vi "DAQ_daqmxorg.vi"() -> ()   [LabVIEW 2020]
uses:
  <vilib>/Utility/error.llb/DialogType.ctl
  <vilib>/DAQmx/read.llb/DAQmx Read (Analog 2D DBL NChan NSamp).vi
  <vilib>/DAQmx/create/channels.llb/DAQmx Create Channel (AI-Voltage-Basic).vi
  <vilib>/DAQmx/configure/timing.llb/DAQmx Timing (Sample Clock).vi
  <vilib>/DAQmx/configure/trigger.llb/DAQmx Start Trigger (None).vi
  <vilib>/DAQmx/miscellaneous.llb/DAQmx Fill In Error Info.vi
panel:
  out "Waveform Chart 2":dbl[][](graph)
  out "data":dbl[][](array[numeric]) format="%0.2f"
  out "Boolean":bool
  in  "stop":bool
  out "Waveform Chart":dbl[][](graph)
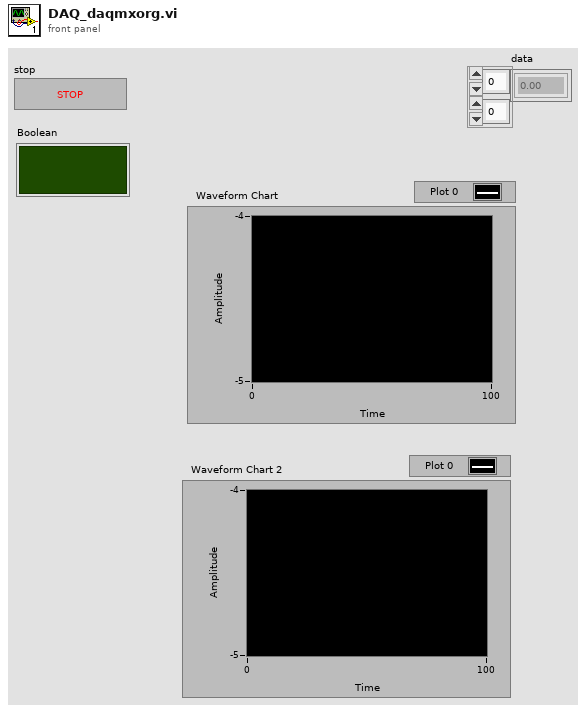
[diagram p1: front panel]
types:
  T1 = typedef "DialogType.ctl" = u16
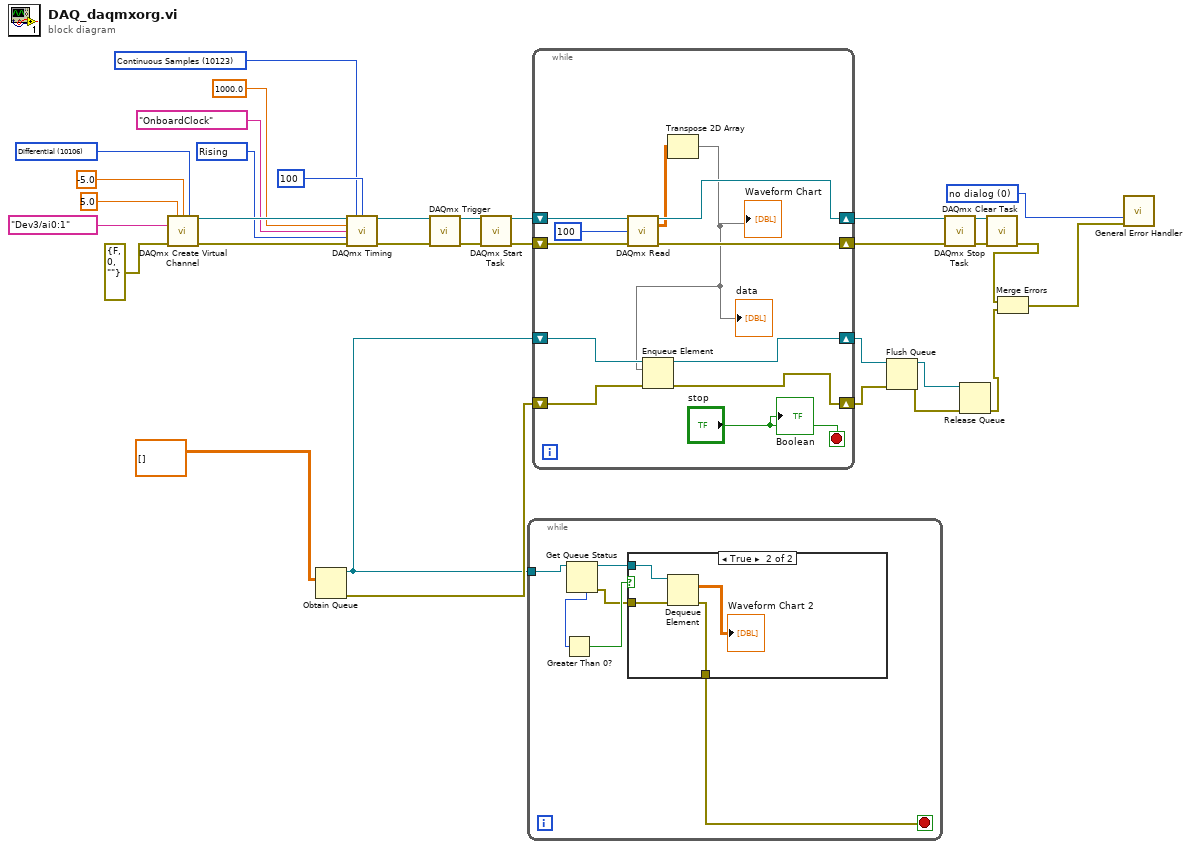
[diagram p0: block diagram]
diagram:
  w11 = T1 0 items=["no dialog", "OK message", "continue or stop message", "OK message + warnings", "continue/stop + warnings"] ("type of dialog (OK msg:1)")
  w22 = 10280 items=["Rising"=10280, "Falling"=10171] ("active edge")
  w25 = 10123 items=["Finite Samples"=10178, "Continuous Samples"=10123, "Hardware Timed Single Point"=12522] ("sample mode")
  w33 = 10106 items=["Default"=-1, "RSE"=10083, "NRSE"=10078, "Differential"=10106, "Pseudodifferential"=12529] ("input terminal configuration")
  n1 = call-poly <vilib>:"DAQmx Create Virtual Channel.vi"("maximum value"=5.0, "minimum value"=-5.0, "input terminal configuration"=w33, "physical channels"=tag "Dev3/ai0:1", "error in"=errorcluster {"status"=FALSE, "code"=0, "source"=""}) -> ("task out"=w27:refnum<k21>, "error out"=w28:errorcluster)  [unwired: 9 in]
  n2 = Obtain Queue(element data type=dbl[][] []) -> (queue out=w6:refnum<queue>, error out=w9:errorcluster)  [unwired: 4 in, 1 out]
  n3 = call-poly <vilib>:"DAQmx Timing.vi"("task/channels in"=w27, "sample mode"=w25, "samples per channel"=100, "rate"=1000.0, "source"=tag "OnboardClock", "active edge"=w22, "error in"=w28) -> ("task out"=w20:refnum<k21>, "error out"=w21:errorcluster)  [unwired: 7 in]
  n4 = call-poly <vilib>:"DAQmx Trigger.vi"("task/channels in"=w20, "error in"=w21) -> ("task out"=w19:refnum<k21>, "error out"=w18:errorcluster)  [unwired: 12 in]
  n5 = call <vilib>:"DAQmx Start Task.vi"("task/channels in"=w19, "error in"=w18) -> ("task out"=w17:refnum<k21>, "error out"=w16:errorcluster)  [unwired: 12 in]
  n6 = while {
    tunnel: w6 -> [w37]
    stop <- w35 stop-if-true
    n7 = Get Queue Status(queue=w37) -> (queue out=w36:refnum<queue>, error out=w34:errorcluster, # elements in queue=w39:i32)  [unwired: 2 in, 5 out]
    n8 = Greater Than 0?(x=w39) -> (x > 0?=w38:bool)
    n9 = case shown="True" w38 {
      tunnel: w36 -> [_ w44]
      tunnel: [w40 w43] -> w35
      tunnel: w34 -> [w40 w42]
      frame False {
      }
      frame True {
        n10 = Dequeue Element(queue=w44, error in (no error)=w42) -> (element=→"Waveform Chart 2":dbl[][], error out=w43:errorcluster)  [unwired: 1 in, 2 out]
      }
    }
  }
  n11 = while {
    shift-right: [w54] -> w15
    shift-left: w17 -> [w56]
    shift-right: [w53] -> w14
    shift-left: w16 -> [w55]
    shift-right: [w47] -> w4
    shift-left: w6 -> [w50]
    shift-right: [w48] -> w2
    shift-left: w9 -> [w49]
    stop <- "stop" stop-if-true
    n12 = call-poly <vilib>:"DAQmx Read.vi"("task/channels in"=w56, "number of samples per channel"=100, "error in"=w55) -> ("task out"=w54:refnum<k21>, "data"=w46:dbl[][], "error out"=w53:errorcluster)  [unwired: 10 in]
    n13 = Transpose 2D Array(2D array=w46) -> (transposed array=w45:dbl[][])
    "Waveform Chart" <- w45
    "data" <- w45
    n14 = Enqueue Element(queue=w50, element=w45, error in (no error)=w49) -> (queue out=w47:refnum<queue>, error out=w48:errorcluster)  [unwired: 1 in, 1 out]
    "Boolean" <- "stop"
  }
  n15 = Flush Queue(queue=w4, error in (no error)=w2) -> (queue out=w3:refnum<queue>, error out=w1:errorcluster)  [unwired: 1 out]
  n16 = call <vilib>:"DAQmx Stop Task.vi"("task/channels in"=w15, "error in"=w14) -> ("task out"=w13:refnum<k21>, "error out"=w12:errorcluster)  [unwired: 12 in]
  n17 = Release Queue(queue=w3, error in (no error)=w1) -> (error out=w5:errorcluster)  [unwired: 1 in, 2 out]
  n18 = call <vilib>:"DAQmx Clear Task.vi"("task in"=w13, "error in"=w12) -> ("error out"=w8:errorcluster)  [unwired: 13 in]
  n19 = Merge Errors(w8, w5) -> (w7:errorcluster)
  n20 = call <vilib>:"General Error Handler.vi"("type of dialog (OK msg:1)"=w11, "error in (no error)"=w7) -> ()  [unwired: 9 in, 5 out]
